vi "Load-Save System Config.vi"(6 "backup file path":path, 7 "Standalone viewer?":bool, 8 "error in":errorcluster, 9 "System Config I/P":T1={"Laser wavelength (nm)"=920.0, "DAQ FPGA System"={"Clock Freq (MHz) "=200.0, "Samples Wait after Trigger"=5080, "AOD fill"=4900, "StartupDelay"=0, "Slip Cycle (clock cycles)"=600000, "Add Cycle"=TRUE}, "Control system"={"AOD 1 Amplitude"=0, "AOD 2 Amplitude"=0, "AOD 3 Amplitude"=0, "AOD 4 Amplitude"=0, "AOD 5 Amplitude"=0, "AOD 6 Amplitude"=0, "T0 (ns)"=0.0, "Ta (ns)"=0.0, "Data Time Interval (ns)"=0.0, "Ctrl FPGA Clock (MHz)"=240.0}} {"Control system"."Ctrl FPGA Clock (MHz)" min=80.0 max=500.0 step=1.0; "Control system"."Data Time Interval (ns)" min=0.0 max=2048.0 step=1.0; "Control system"."Ta (ns)" min=0.0 max=2048.0 step=1.0; "Control system"."T0 (ns)" min=0.0 max=2048.0 step=1.0; "Control system"."AOD 6 Amplitude" min=0 max=2048 step=1; "Control system"."AOD 5 Amplitude" min=0 max=2048 step=1; "Control system"."AOD 4 Amplitude" min=0 max=2048 step=1; "Control system"."AOD 3 Amplitude" min=0 max=2048 step=1; "Control system"."AOD 2 Amplitude" min=0 max=2048 step=1; "Control system"."AOD 1 Amplitude" min=0 max=2048 step=1; "Laser wavelength (nm)" min=800.0 max=1080.0 step=1.0}, 11 "Function":T4=enum."Load from file") -> (0 "error out":errorcluster, 1 "System Config O/P":T1={"Laser wavelength (nm)"=920.0, "DAQ FPGA System"={"Clock Freq (MHz) "=200.0, "Samples Wait after Trigger"=5080, "AOD fill"=4900, "StartupDelay"=0, "Slip Cycle (clock cycles)"=600000, "Add Cycle"=TRUE}, "Control system"={"AOD 1 Amplitude"=0, "AOD 2 Amplitude"=0, "AOD 3 Amplitude"=0, "AOD 4 Amplitude"=0, "AOD 5 Amplitude"=0, "AOD 6 Amplitude"=0, "T0 (ns)"=0.0, "Ta (ns)"=0.0, "Data Time Interval (ns)"=0.0, "Ctrl FPGA Clock (MHz)"=240.0}} {"Control system"."Ctrl FPGA Clock (MHz)" min=80.0 max=500.0 step=1.0; "Control system"."Data Time Interval (ns)" min=0.0 max=2048.0 step=1.0; "Control system"."Ta (ns)" min=0.0 max=2048.0 step=1.0; "Control system"."T0 (ns)" min=0.0 max=2048.0 step=1.0; "Control system"."AOD 6 Amplitude" min=0 max=2048 step=1; "Control system"."AOD 5 Amplitude" min=0 max=2048 step=1; "Control system"."AOD 4 Amplitude" min=0 max=2048 step=1; "Control system"."AOD 3 Amplitude" min=0 max=2048 step=1; "Control system"."AOD 2 Amplitude" min=0 max=2048 step=1; "Control system"."AOD 1 Amplitude" min=0 max=2048 step=1; "Laser wavelength (nm)" min=800.0 max=1080.0 step=1.0})   [LabVIEW 2020]
uses:
  Typedefs/Save-Load enum.ctl
  Typedefs/System Configuration.ctl
  Typedefs/DAQ FPGA system config.ctl
  Typedefs/CTRL system config.ctl
  Typedefs/Which path.ctl
  <vilib>/Utility/config.llb/NI_LVConfig.lvlib
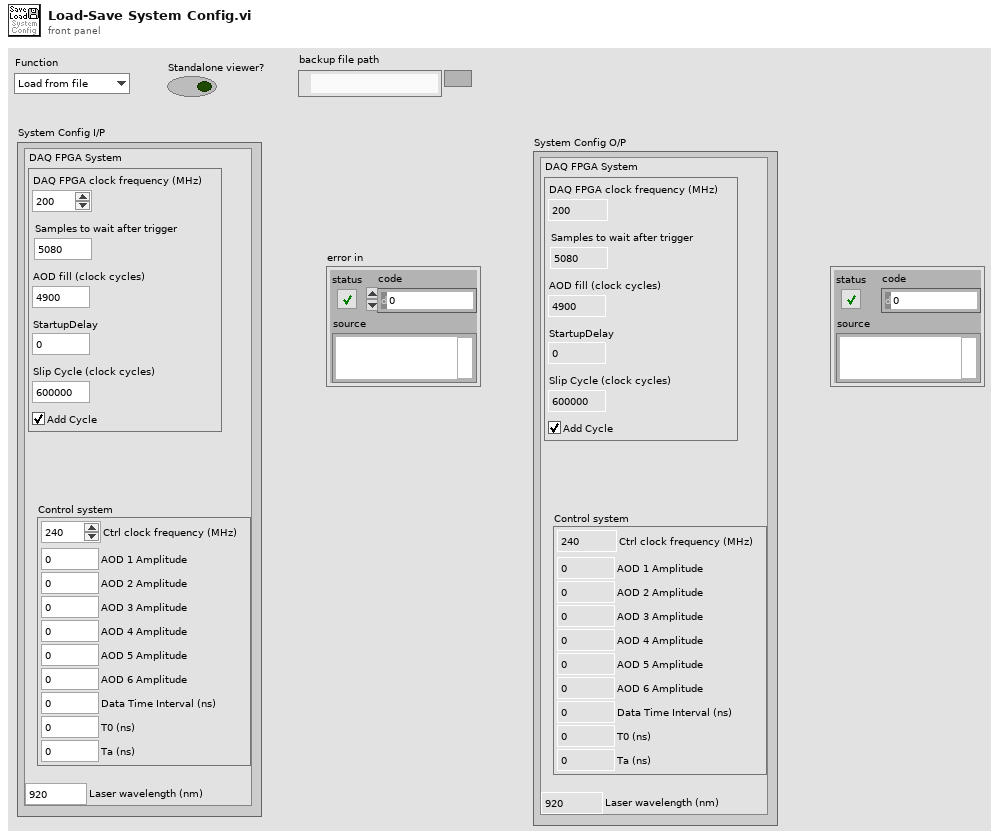
[diagram p1: front panel]
types:
  T1 = typedef "System Configuration.ctl" = cluster{"Laser wavelength (nm)":dbl, "DAQ FPGA System":T2, "Control system":T3}
  T2 = typedef "DAQ FPGA system config.ctl" = cluster{"Clock Freq (MHz) ":dbl, "Samples Wait after Trigger":u16, "AOD fill":u16, "StartupDelay":i32, "Slip Cycle (clock cycles)":u32, "Add Cycle":bool}
  T3 = typedef "CTRL system config.ctl" = cluster{"AOD 1 Amplitude":i16, "AOD 2 Amplitude":i16, "AOD 3 Amplitude":i16, "AOD 4 Amplitude":i16, "AOD 5 Amplitude":i16, "AOD 6 Amplitude":i16, "T0 (ns)":dbl, "Ta (ns)":dbl, "Data Time Interval (ns)":dbl, "Ctrl FPGA Clock (MHz)":dbl}
  T4 = typedef "Save-Load enum.ctl" = enum16{"Save to file", "Load from file", "Compare from file", "Save Backup"}
  T5 = typedef "Which path.ctl" = enum16{"Configuration Files", "Calibration Files", "Images", "Setup.ini", "Loaded User profile.ini", "User's-Previous session.ini", "New user profile.ini", "Selected User profile.ini", "User profiles folder", "Power meter scaling.txt", "FOV Cal.ini", "Calibration.ini"}
  T6 = typedef "NI_LVConfig.lvlib/Config Data RefNum.ctl" = refnum<k1>
  T7 = cluster{"key":string, "Save?":bool, "Default":string}[]
  T8 = typedef "Ini file interface (DBL).ctl" = cluster{"key":string, "Save?":bool, "Default":dbl}[]
  T9 = cluster{"key":string, "Save?":bool, "Default":bool}[]
  T10 = cluster{"key":string, "Save?":bool, "Default":dbl}
  T11 = cluster{"key":string, "Save?":bool, "Default":dbl}[]
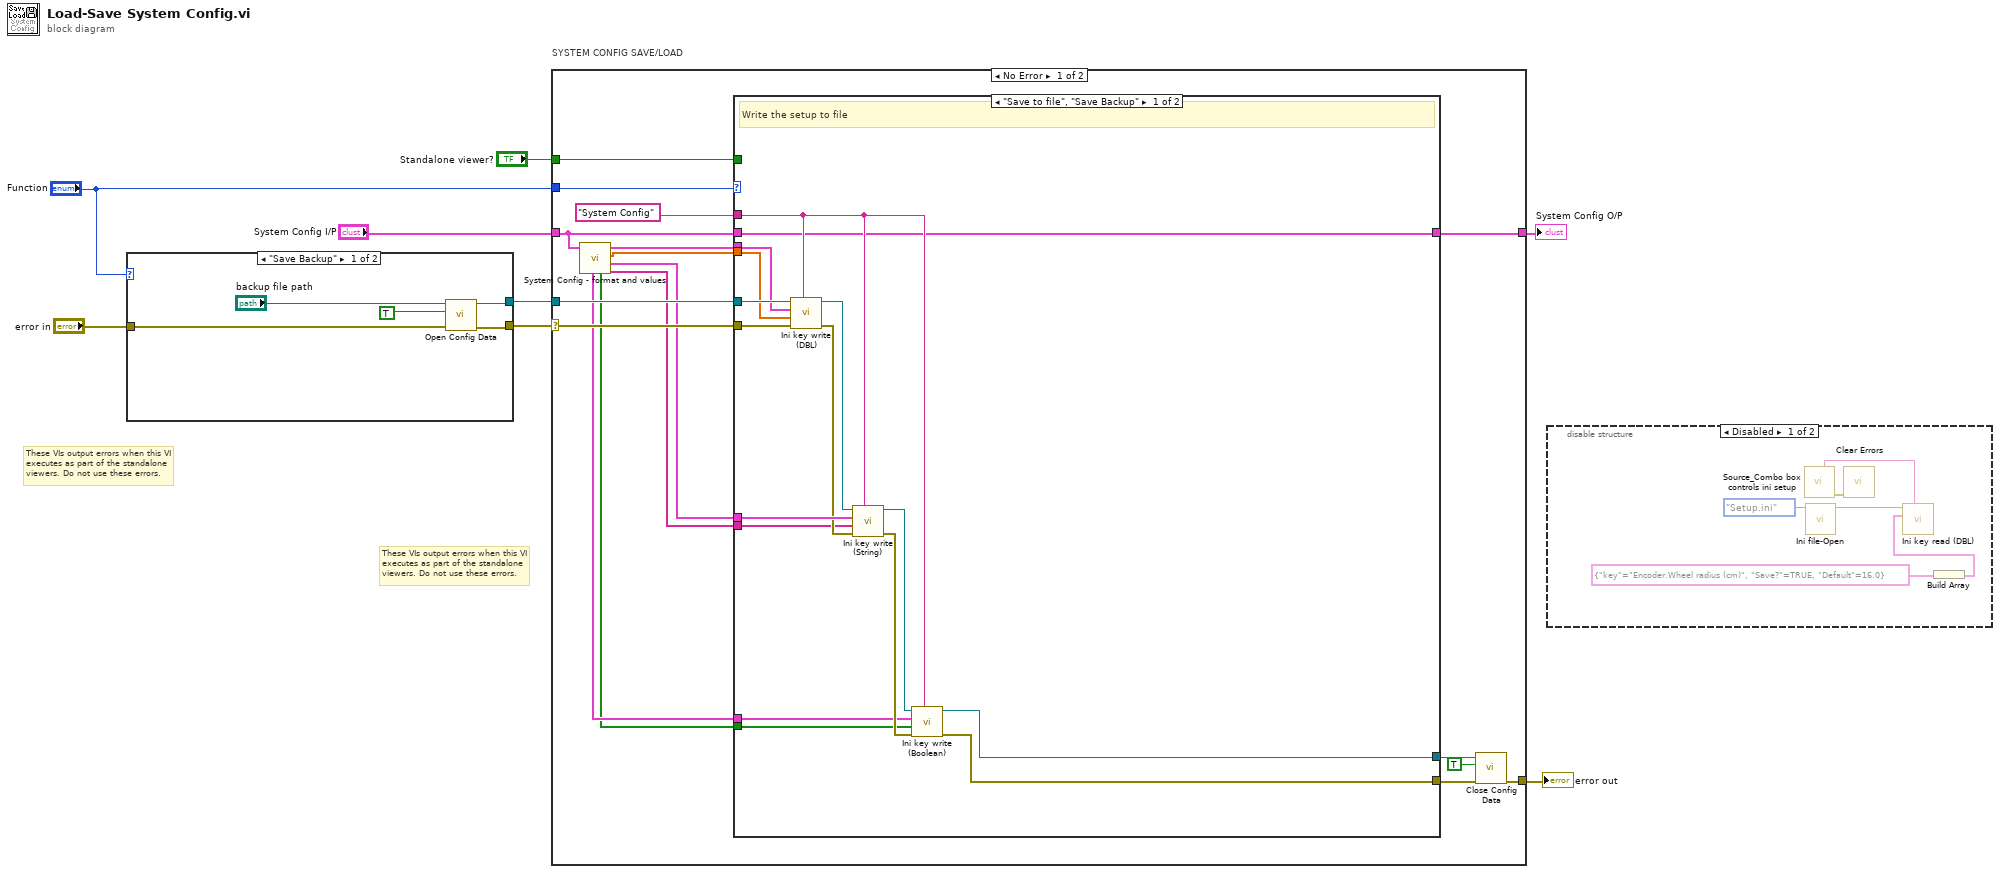
[diagram p0: block diagram]
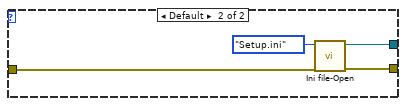
[diagram p2: hidden frame]
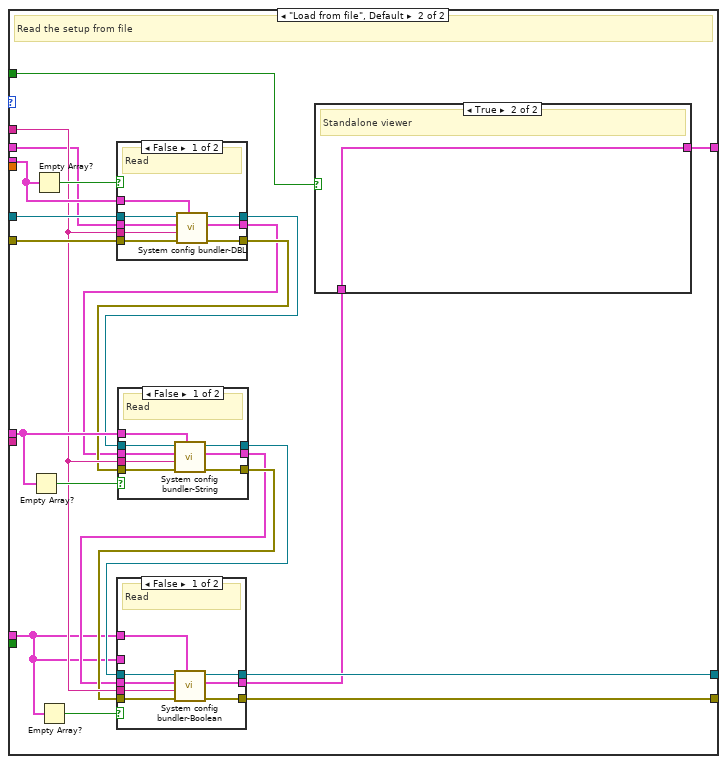
[diagram p4: hidden frame]
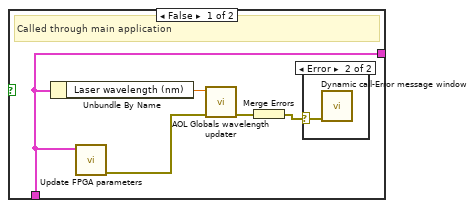
[diagram p5: hidden frame]
diagram:
  # "These VIs output errors when this VI executes as part of the standalone viewers. Do not use these errors."
  # "These VIs output errors when this VI executes as part of the standalone viewers. Do not use these errors."
  n1 = case shown="\"Save Backup\"" "Function" {
    tunnel: [w10 w16] -> w8
    tunnel: [w11 w15] -> w7
    tunnel: "error in" -> [w12 w14]
    frame "Save Backup" {
      n2 = call <vilib>:"Open Config Data.vi"("error in (no error)"=w12, "create file if necessary (T)"=TRUE ("create file if necessary"), "configuration file path"="backup file path") -> ("error out"=w10:errorcluster, "refnum"=w11:T6)  [unwired: 6 in, 1 out]
    }
    frame Default {
      n3 = call "Ini file-Open.vi"("Error In"=w14, "Which file?"=Which_path."Setup.ini") -> ("error out"=w16:errorcluster, "User profile ini file ref"=w15:T6)  [unwired: 6 in, 2 out]
    }
  }
  n4 = case "SYSTEM CONFIG SAVE/LOAD" shown="No Error" w8 {
    selector: w8 -> [w30 w113]
    tunnel: [w28 w113] -> w6
    tunnel: "System Config I/P" -> [w24 w112]
    tunnel: [w32 w112] -> w3
    tunnel: "Function" -> [w31 _]
    tunnel: w7 -> [w29 _]
    tunnel: "Standalone viewer?" -> [w26 _]
    frame No Error {
      n5 = call "System Config - format and values.vi"("System Config"=w24) -> ("String Values"=w21:string[], "String"=w22:T7, "Numeric Values"=w23:dbl[], "Numeric"=w25:T8, "Boolean Values"=w19:bool[], "Boolean"=w20:T9)  [unwired: 5 in]
      n6 = case shown="\"Save to file\", \"Save Backup\"" w31 {
        tunnel: [w39 w66] -> w27
        tunnel: [w38 w67] -> w33
        tunnel: w30 -> [w49 w68]
        tunnel: w29 -> [w50 w71]
        tunnel: "System Config" ("key") -> [w40 w62]
        tunnel: w25 -> [w47 w70]
        tunnel: w23 -> [w48 _]
        tunnel: w21 -> [w43 _]
        tunnel: w22 -> [w46 w63]
        tunnel: [w37 w54] -> w32
        tunnel: w24 -> [w37 w57]
        tunnel: w26 -> [_ w52]
        tunnel: w20 -> [w36 w51]
        tunnel: w19 -> [w35 _]
        frame "Save to file", "Save Backup" {
          # "Write the setup to file"
          n7 = call "Ini key write (DBL).vi"("Section"=w40, "error in (no error)"=w49, "Values (DBL)"=w48, "Ini file interface"=w47, "Ini file refnum in"=w50) -> ("error out"=w44:errorcluster, "Ini file refnum out"=w45:T6)  [unwired: 5 in]
          n8 = call "Ini key write (String).vi"("Section"=w40, "error in (no error)"=w44, "Values (String)"=w43, "Ini file interface"=w46, "Ini file refnum in"=w45) -> ("error out"=w41:errorcluster, "Ini file refnum out"=w42:T6)  [unwired: 5 in]
          n9 = call "Ini key write (Boolean).vi"("Section"=w40, "error in (no error)"=w41, "Values (Boolean)"=w35, "Ini file interface"=w36, "Ini file refnum in"=w42) -> ("error out"=w39:errorcluster, "Ini file refnum out"=w38:T6)  [unwired: 5 in]
        }
        frame "Load from file", Default {
          # "Read the setup from file"
          n10 = Empty Array?(array=w63) -> (empty?=w64:bool)
          n11 = Empty Array?(array=w70) -> (empty?=w69:bool)
          n12 = Empty Array?(array=w51) -> (empty?=w65:bool)
          n13 = case shown="False" w69 {
            tunnel: w71 -> [w108 w111]
            tunnel: [w107 w111] -> w58
            tunnel: [w106 w110] -> w59
            tunnel: w68 -> [w105 w110]
            tunnel: w62 -> [w103 _]
            tunnel: w70 -> [w104 _]
            tunnel: w57 -> [w101 w109]
            tunnel: [w102 w109] -> w56
            frame False {
              # "Read"
              n14 = call "System config bundler-DBL.vi"("Keys setup.DBL"=w104, "error in (no error)"=w105, "Section name"=w103, "System Config I/P"=w101, "Refnum in"=w108) -> ("error out"=w106:errorcluster, "System Config O/P"=w102:T1, "Refnum out"=w107:T6)  [unwired: 4 in]
            }
            frame True {
              # "No parametersof such type"
            }
          }
          n15 = case shown="False" w64 {
            tunnel: [w84 w89] -> w61
            tunnel: [w83 w88] -> w60
            tunnel: w63 -> [w79 _]
            tunnel: w58 -> [w86 w89]
            tunnel: w59 -> [w82 w88]
            tunnel: w62 -> [w85 _]
            tunnel: w56 -> [w80 w87]
            tunnel: [w81 w87] -> w55
            frame False {
              # "Read"
              n16 = call "System config bundler-String.vi"("Keys setup.String"=w79, "error in (no error)"=w82, "Section name"=w85, "System Config I/P"=w80, "Refnum in"=w86) -> ("error out"=w83:errorcluster, "System Config O/P"=w81:T1, "Refnum out"=w84:T6)  [unwired: 4 in]
            }
            frame True {
              # "No parametersof such type"
            }
          }
          n17 = case shown="False" w65 {
            tunnel: [w96 w100] -> w67
            tunnel: [w95 w99] -> w66
            tunnel: w51 -> [_ _]
            tunnel: w61 -> [w97 w100]
            tunnel: w60 -> [w94 w99]
            tunnel: w62 -> [w93 _]
            tunnel: w55 -> [w90 w98]
            tunnel: [w92 w98] -> w53
            tunnel: w51 -> [w91 _]
            frame False {
              # "Read"
              n18 = call "System config bundler-Boolean.vi"("Keys setup.Boolean"=w91, "error in (no error)"=w94, "Section name"=w93, "System Config I/P"=w90, "Refnum in"=w97) -> ("error out"=w95:errorcluster, "System Config I/P"=w92:T1, "Refnum out"=w96:T6)  [unwired: 4 in]
            }
            frame True {
              # "No parametersof such type"
            }
          }
          n19 = case shown="True" w52 {
            tunnel: [w75 w78] -> w54
            tunnel: w53 -> [w75 w78]
            frame False {
              # "Called through main application"
              n20 = Unbundle By Name(w75) -> ("Laser wavelength (nm)"=w76:dbl)
              n21 = call "Update FPGA parameters.vi"("System Config I/P"=w75) -> ("error out"=w72:errorcluster)  [unwired: 10 in]
              n22 = call "AOL Globals wavelength updater.vi"("error in (no error)"=w72, "Laser wavelength (nm)"=w76) -> ("error out"=w74:errorcluster)  [unwired: 9 in]
              n23 = Merge Errors(w74) -> (w73:errorcluster)
              n24 = case shown="Error" w73 {
                selector: w73 -> [_ w77]
                frame No Error {
                }
                frame Error {
                  n25 = call "Dynamic call-Error message window.vi"("error in (no error)"=w77) -> ()  [unwired: 10 in, 1 out]
                }
              }
            }
            frame True {
              # "Standalone viewer"
            }
          }
        }
      }
      n26 = call <vilib>:"Close Config Data.vi"("error in (no error)"=w27, "write file if changed (T)"=TRUE ("write configuration file? (F)"), "refnum"=w33) -> ("error out"=w28:errorcluster)  [unwired: 7 in, 1 out]
    }
    frame Error {
    }
  }
  "error out" <- w6
  "System Config O/P" <- w3
  n27 = disable-structure shown="Disabled" {
    frame Disabled {
      n28 = call "Source_Combo box controls ini setup.vi"() -> ("error out"=w114:errorcluster, "Section name"=w115:string)  [unwired: 9 in, 1 out]
      n29 = call "Ini file-Open.vi"("Which file?"=Which_path."Setup.ini") -> ("User profile ini file ref"=w118:T6)  [unwired: 7 in, 3 out]
      n30 = call <vilib>:"Clear Errors.vi"("error in (no error)"=w114) -> ()  [unwired: 5 in, 2 out]
      n31 = Build Array(T10 {"key"="Encoder.Wheel radius (cm)", "Save?"=TRUE, "Default"=16.0}) -> (w116:T11)
      n32 = call "Ini key read (DBL).vi"("Section name"=w115, "Parameter names & setup"=w116, "Ini file refnum in"=w118) -> ()  [unwired: 6 in, 3 out]
    }
    frame Enabled {
    }
  }
